vi "EncodeInt64.vi"(1 "Data In":i64[](array[numeric])) -> (0 "Data Out":u8[](array[numeric]))   [LabVIEW 2014, in "navX-MXP IMU.lvlib"]
uses:
  navX-MXP IMU.lvlib
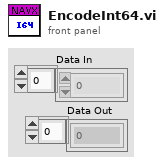
[diagram p1: front panel]
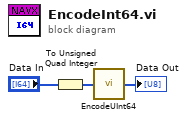
[diagram p0: block diagram]
diagram:
  n1 = To Unsigned Quad Integer(1:"Data In") -> (0:w2:u64[])
  n2 = call "EncodeUInt64.vi"("Data In"=w2) -> ("Data Out"=→"Data Out":u8[])
